vi "VI Tree.vi"   [LabVIEW 2012, in "TDK-Lambda Z.lvlib"]
doc: "This is the instrument driver for the TDK-Lambda Z+ Series. The VI Tree displays all the user-callable VIs of the instrument driver in an organized table."
uses:
  TDK-Lambda Z.lvlib
  Configure/Trigger/Configure Trigger (Current).vi
  Configure/Waveform/Configure Waveform (Voltage).vi
  Configure/List/Configure List (Voltage).vi
  Action-Status/Transient Memory (Load).vi
panel:
  # "(c) 2014-2015 TDK-Lambda.  ALL RIGHTS RESERVED."
  # "SEE DIAGRAM\nFOR VI TREE."
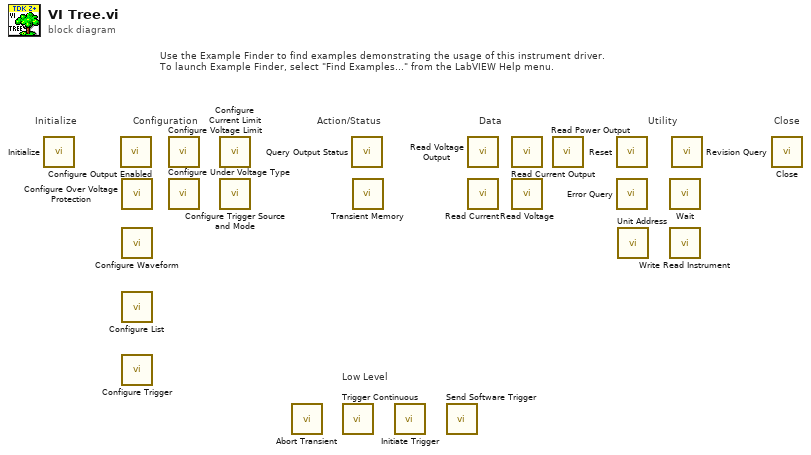
[diagram p0: block diagram]
diagram:
  # "Low Level"
  # "Use the Example Finder to find examples demonstrating the usage of this instrument driver.\nTo launch Example Finder, select \"Find Examples...\" from the LabVIEW Help menu."
  # "Configuration"
  # "Utility"
  # "Data"
  # "Action/Status"
  # "Close"
  # "Initialize"
  n1 = call "Initialize.vi"() -> ()  [unwired: 10 in, 2 out]
  n2 = call "Configure Output Enabled.vi"() -> ()  [unwired: 10 in, 2 out]
  n3 = call "Configure Over Voltage Protection.vi"() -> ()  [unwired: 10 in, 2 out]
  n4 = call-poly "Configure Waveform.vi"() -> ()  [unwired: 10 in, 2 out]
  n5 = call-poly "Configure List.vi"() -> ()  [unwired: 10 in, 2 out]
  n6 = call-poly "Configure Trigger.vi"() -> ()  [unwired: 10 in, 2 out]
  n7 = call "Configure Voltage Limit.vi"() -> ()  [unwired: 10 in, 2 out]
  n8 = call "Configure Under Voltage Type.vi"() -> ()  [unwired: 10 in, 2 out]
  n9 = call "Configure Current Limit.vi"() -> ()  [unwired: 10 in, 2 out]
  n10 = call "Configure Trigger Source and Mode.vi"() -> ()  [unwired: 10 in, 2 out]
  n11 = call "Abort Transient.vi"() -> ()  [unwired: 10 in, 2 out]
  n12 = call "Trigger Continuous.vi"() -> ()  [unwired: 10 in, 2 out]
  n13 = call "Query Output Status.vi"() -> ()  [unwired: 9 in, 3 out]
  n14 = call-poly "Transient Memory.vi"() -> ()  [unwired: 10 in, 2 out]
  n15 = call "Initiate Trigger.vi"() -> ()  [unwired: 10 in, 2 out]
  n16 = call "Send Software Trigger.vi"() -> ()  [unwired: 10 in, 2 out]
  n17 = call "Read Voltage Output .vi"() -> ()  [unwired: 9 in, 3 out]
  n18 = call "Read Current.vi"() -> ()  [unwired: 9 in, 3 out]
  n19 = call "Read Current Output.vi"() -> ()  [unwired: 9 in, 3 out]
  n20 = call "Read Voltage.vi"() -> ()  [unwired: 9 in, 3 out]
  n21 = call "Read Power Output.vi"() -> ()  [unwired: 9 in, 3 out]
  n22 = call "Reset.vi"() -> ()  [unwired: 10 in, 2 out]
  n23 = call "Error Query.vi"() -> ()  [unwired: 8 in, 4 out]
  n24 = call "Unit Address.vi"() -> ()  [unwired: 10 in, 2 out]
  n25 = call "Wait.vi"() -> ()  [unwired: 10 in, 2 out]
  n26 = call "Write Read Instrument.vi"() -> ()  [unwired: 9 in, 3 out]
  n27 = call "Revision Query.vi"() -> ()  [unwired: 8 in, 4 out]
  n28 = call "Close.vi"() -> ()  [unwired: 11 in, 1 out]
